vi "Get Home Search Mode.vi"(4 "error in (no error)":errorcluster, 6 "Axis (1)":i32=1 min=1 max=3, 7 "VISA resource name":refnum<visa-resource-name>) -> (0 "error out":errorcluster, 2 "Home search mode":T1(ring), 3 "VISA resource name out":refnum<visa-resource-name>)   [LabVIEW 2012, in "Newport ESP301.lvlib"]
doc: "Reads the Home search mode invoking in the home search sequence on the specified axis.\n\nThe \"home search mode\" parameter is overwritten by the \"Search For Home.vi\" command parameter."
uses:
  Newport ESP301.lvlib
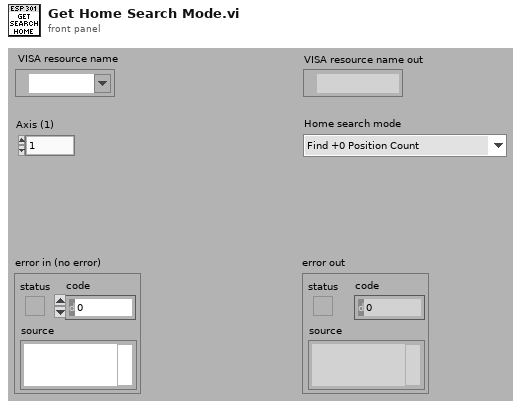
[diagram p1: front panel]
types:
  T1 = enum16{"Find +0 Position Count", "Find Home and Index Signals", "Find Home Signal", "Find Positive Limit Signal", "Find Negative Limit Signal", "Find Positve Limit and Index Signals", "Find Negative Limit and Index Signals"}
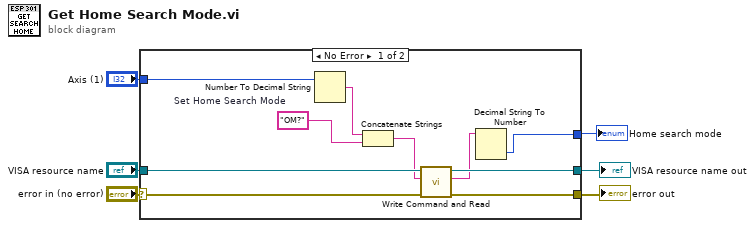
[diagram p0: block diagram]
diagram:
  n1 = case shown="No Error" "error in (no error)" {
    selector: "error in (no error)" -> [w15 w18]
    tunnel: [w14 w18] -> w5
    tunnel: "VISA resource name" -> [w16 w17]
    tunnel: [w13 w17] -> w3
    tunnel: "Axis (1)" -> [w10 _]
    tunnel: [w7 _] -> w1
    frame No Error {
      w12 = "OM?"  # Set Home Search Mode
      n2 = Number To Decimal String(number=w10) -> (decimal integer string=w11:string)  [unwired: 1 in]
      n3 = Concatenate Strings(w11, w12) -> (w9:string)
      n4 = call "Write Command and Read.vi"("error in (no error)"=w15, "Command"=w9, "VISA resource name"=w16) -> ("error out"=w14:errorcluster, "Returned string"=w8:string, "VISA resource name out"=w13:refnum<visa-resource-name>)  [unwired: 4 in]
      n5 = Decimal String To Number(string=w8) -> (number=w7:i32)  [unwired: 2 in, 1 out]
    }
    frame Error {
    }
  }
  "error out" <- w5
  "VISA resource name out" <- w3
  "Home search mode" <- w1
